vi "MT_Open.vi"(8 "Error In":errorcluster caption="错误输入") -> (0 "Error Out":errorcluster caption="错误输出", 3 "MT设备状态":bool)   [LabVIEW 2020]
uses:
  lib/MT/MT_API.lvlib
panel:
  # "打开MT设备"
  # "设备打开状态"
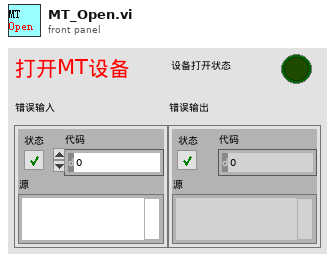
[diagram p1: front panel]
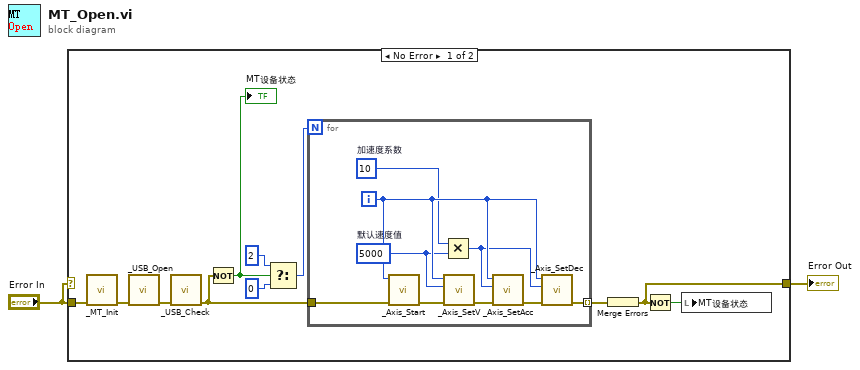
[diagram p0: block diagram]
diagram:
  n1 = case shown="No Error" "Error In" {
    selector: "Error In" -> [_ w23]
    tunnel: [w12 w23] -> w2
    tunnel: "Error In" -> [w9 _]
    frame No Error {
      n2 = call "_MT_Init.vi"("Error In"=w9) -> ("Error Out"=w11:errorcluster)  [unwired: 10 in]
      n3 = call "_USB_Open.vi"("Error In"=w11) -> ("Error Out"=w10:errorcluster)  [unwired: 10 in]
      n4 = call "_USB_Check.vi"("Error In"=w10) -> ("Error Out"=w8:errorcluster)  [unwired: 10 in]
      n5 = Not(x=w8) -> (.not. x?=w13:bool)
      "MT设备状态" <- w13
      n6 = Select(t=2, s=w13, f=0) -> (s? t:f=w7:i32)
      n7 = for {
        N: w7 -> [_]
        tunnel: w8 -> [w21]
        tunnel: [w18] -> w4 mode=indexing
        i -> [w22]
        w14 = 10  # 加速度系数
        w15 = 5000  # 默认速度值
        n8 = call "_Axis_Start.vi"("Error In"=w21, "轴序号"=w22) -> ("Error Out"=w20:errorcluster)  [unwired: 9 in]
        n9 = Multiply(x=w14, y=w15) -> (x*y=w16:i32)
        n10 = call "_Axis_SetV.vi"("Error In"=w20, "最大速度"=w15, "轴序号"=w22) -> ("Error Out"=w19:errorcluster)  [unwired: 8 in]
        n11 = call "_Axis_SetAcc.vi"("Error In"=w19, "加速度值"=w16, "轴序号"=w22) -> ("Error Out"=w17:errorcluster)  [unwired: 8 in]
        n12 = call "_Axis_SetDec.vi"("Error In"=w17, "减速度值"=w16, "轴序号"=w22) -> ("Error Out"=w18:errorcluster)  [unwired: 8 in]
      }
      n13 = Merge Errors(w4) -> (w12:errorcluster)
      n14 = Not(x=w12) -> (.not. x?=w3:bool)
      n15 = local write "MT设备状态"(w3) -> ()
    }
    frame Error {
    }
  }
  "Error Out" <- w2
